vi "Array.vi"() -> ()   [LabVIEW 2018]
panel:
  in  "2차원 배열":bool[][](array[boolean])
  in  "1차원 배열":dbl[](array[numeric])
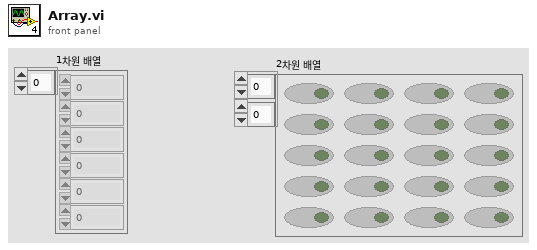
[diagram p1: front panel]
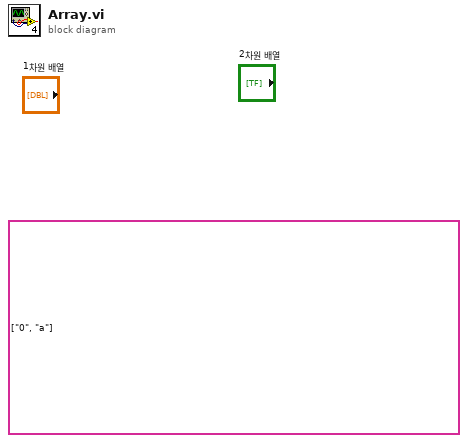
[diagram p0: block diagram]
diagram:
  (unwired) string[][] [["0"], ["a"]]
